vi "get_uMp_version.vi"(8 "error in (no error)":errorcluster, 11 "Handle in":i64) -> (0 "error out":errorcluster, 1 "uMp version":i32[](array[numeric]), 2 "Return (<0 is error)":i32, 3 "Handle out":i64)   [LabVIEW 2016, in "OSB_uMp_library.lvlib"]
doc: "Returns version number for uMp."
uses:
  OSB_uMp_library.lvlib
  ump.dll
panel:
  # "By Stuart Box at OxSyBio Ltd, 2017\n\nThis software is provided WITHOUT ANY WARRANTY; without even the implied warranty of MERCHANTABILITY or FITNESS FOR A PARTICULAR PURPOSE.\n\ninfo@oxsybio.com\n\nOxSyBio Ltd, The Walbrook Building, 25 Walbrook, London, EC4N 8AF"
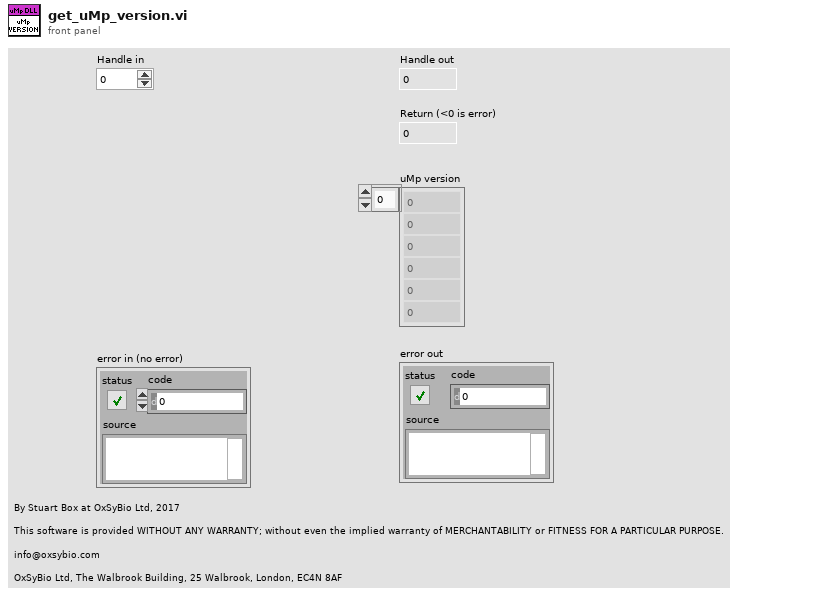
[diagram p1: front panel]
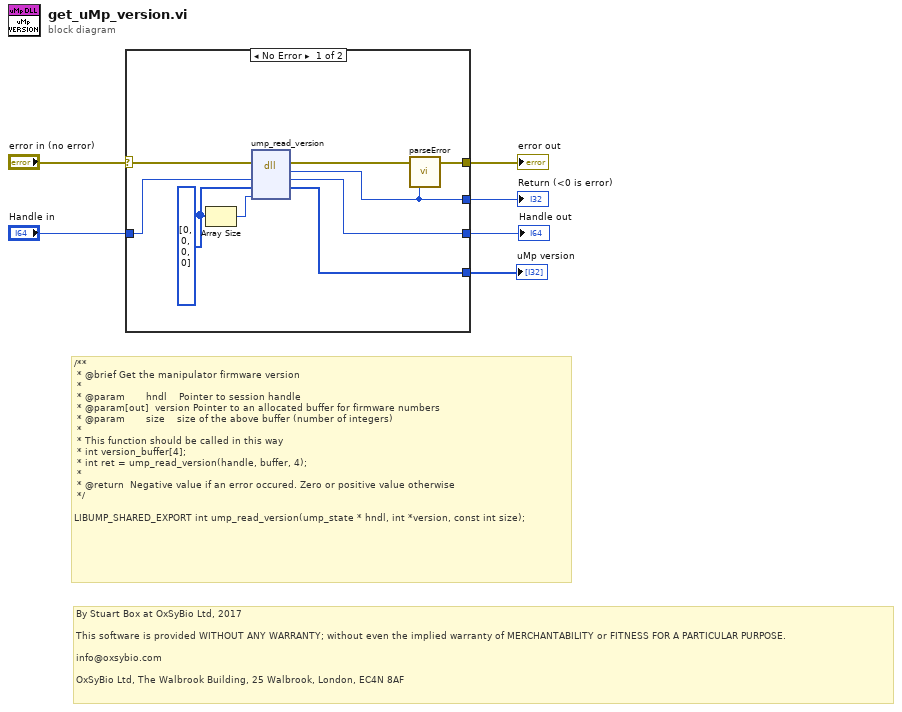
[diagram p0: block diagram]
diagram:
  # "By Stuart Box at OxSyBio Ltd, 2017\n\nThis software is provided WITHOUT ANY WARRANTY; without even the implied warranty of MERCHANTABILITY or FITNESS FOR A PARTICULAR PURPOSE.\n\ninfo@oxsybio.com\n\nOxSyBio Ltd, The Walbrook Building, 25 Walbrook, London, EC4N 8AF"
  # "/**\n * @brief Get the manipulator firmware version\n *\n * @param       hndl    Pointer to session handle\n * @param[out]  version Pointer to an allocated buffer for firmware numbers\n * @param       size    size of the above buffer (number of integers)\n *\n * This function should be called in this way\n * int version_buffer[4];\n * int ret = ump_read_version(handle, buffer, 4);\n *\n * @return  Negative value if an error occured. Zero or positive value otherwise\n */\n\nLIBUMP_SHARED_EXPORT int ump_read_version(ump_state * hndl, int *version, const int size);"
  n1 = case shown="No Error" "error in (no error)" {
    selector: "error in (no error)" -> [w13 w17]
    tunnel: "Handle in" -> [w12 w16]
    tunnel: [w8 w17] -> w5
    tunnel: [w7 _] -> w4
    tunnel: [w11 w16] -> w3
    tunnel: [w10 _] -> w1
    frame No Error {
      w15 = i32[] [0, 0, 0, 0] ("version")
      n2 = Array Size(array=w15) -> (size(s)=w14:i32)
      n3 = dll-call lib="C:/Users/Stu/Desktop/OSB LabVIEW uMp/uMp_library/ump.dll" fn="ump_read_version"(error in=w13, "handle"=w12, "version"=w15, "size"=w14) -> (error out=w9:errorcluster, "return"=w7:i32, "handle"=w11:i64, "version"=w10:i32[])  [unwired: 3 in, 1 out]
      n4 = call "parseError.vi"("Error In"=w9, "ump dll return value (<0 is error)"=w7) -> ("Error Out"=w8:errorcluster)  [unwired: 24 in, 1 out]
    }
    frame Error {
    }
  }
  "error out" <- w5
  "Return (<0 is error)" <- w4
  "Handle out" <- w3
  "uMp version" <- w1
